vi "Cleanup Session.vi"(8 "error in":errorcluster, 11 "Plugin in":refnum<class "DFT_Spectra.lvclass">) -> (0 "error out":errorcluster, 3 "Plugin out":refnum<class "DFT_Spectra.lvclass">)   [LabVIEW 2023, in "DFT_Spectra.lvlib" / "DFT_Spectra.lvclass"]
uses:
  DFT_Spectra.lvclass
  DFT_Spectra.lvclass/DFT_Spectra.ctl
  <vilib>/addons/_NISVFA/_Shared subVIs/Data Objects/Waveforms (DBL)/Waveforms (N Ch).lvclass
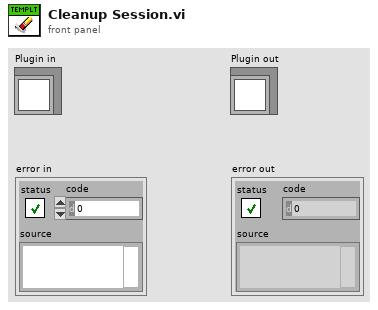
[diagram p1: front panel]
types:
  T1 = enum32{"Invalid", "Standard", "Closed", "Hidden", "Minimized", "Maximized"}
  T2 = typedef "DFT_Spectra.lvlib/DFT_Spectra.lvclass/Power Spectrum Density Data.ctl" = cluster{"First Time":bool, "Show Results Window":bool, "Show Results Window Clicked":bool, "Window":T3, "overlap":i32, "Block Duration":dbl, "Averaging parameters":cluster{"averaging mode":enum16{"No averaging", "Vector averaging", "RMS averaging", "Peak hold"}, "weighting mode":enum16{"Linear", "Exponential"}, "number of averages":u32}, "Spectra UI":refnum<vi>, "buffer out":refnum<data-value>}
  T3 = typedef "NI_AALPro.lvlib/windowTd.ctl" = u32
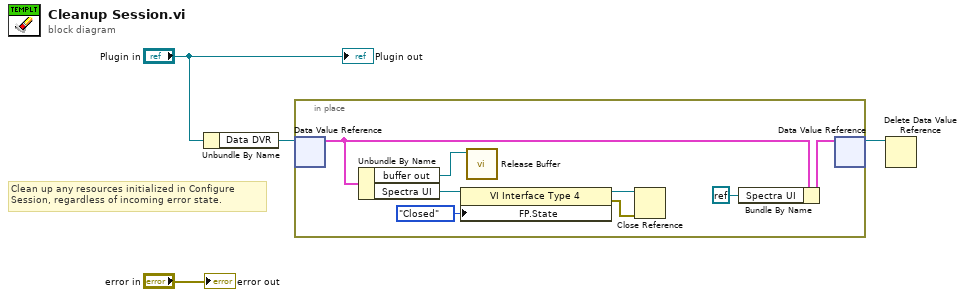
[diagram p0: block diagram]
diagram:
  # "Clean up any resources initialized in Configure Session, regardless of incoming error state."
  n1 = Unbundle By Name("Plugin in") -> ("Data DVR"=w4:refnum<data-value>)
  n2 = in-place {
    n3 = in-place-dvr #1(w4) -> (w12:T2)  [unwired: 1 out]
    n4 = Unbundle By Name(w12) -> ("buffer out"=w5:refnum<data-value>, "Spectra UI"=w10:refnum<vi>)
    n5 = property class="VI Interface Type 4"(reference=w10, "FP.State"=T1."Closed" ("Front Panel Window:State")) -> (reference out=w9:refnum<vi>, error out=w7:errorcluster)  [unwired: 1 in]
    n6 = call <vilib>:"Release Buffer.vi"("buffer"=w5) -> ()  [unwired: 10 in, 1 out]
    n7 = Close Reference(reference=w9, error in (no error)=w7) -> ()  [unwired: 1 out]
    n8 = Bundle By Name(cluster=w12, "Spectra UI"=refnum<k0> refnum) -> (w6:T2)
    n9 = in-place-dvr #1(w6) -> (w3:refnum<data-value>)  [unwired: 1 out]
  }
  n10 = Delete Data Value Reference(data value reference=w3) -> ()  [unwired: 1 in, 2 out]
  "error out" <- "error in"
  "Plugin out" <- "Plugin in"
